vi "Joystick 0 Solenoids.vi"(8 "error in (no error)":errorcluster, 11 "button value":bool) -> (0 "error out":errorcluster)   [LabVIEW 2015]
uses:
  <vilib>/Rock Robotics/WPI/Solenoid/WPI_SolenoidValue.ctl
  <vilib>/Rock Robotics/WPI/Solenoid/Deprecated/WPI_SolenoidGetBool.vi
  <vilib>/Rock Robotics/WPI/Solenoid/WPI_SolenoidSetEnum.vi
panel:
  in  "button value 2":bool
  out "error out 2":errorcluster
  in  "error in (no error) 2":errorcluster
  # "ee"
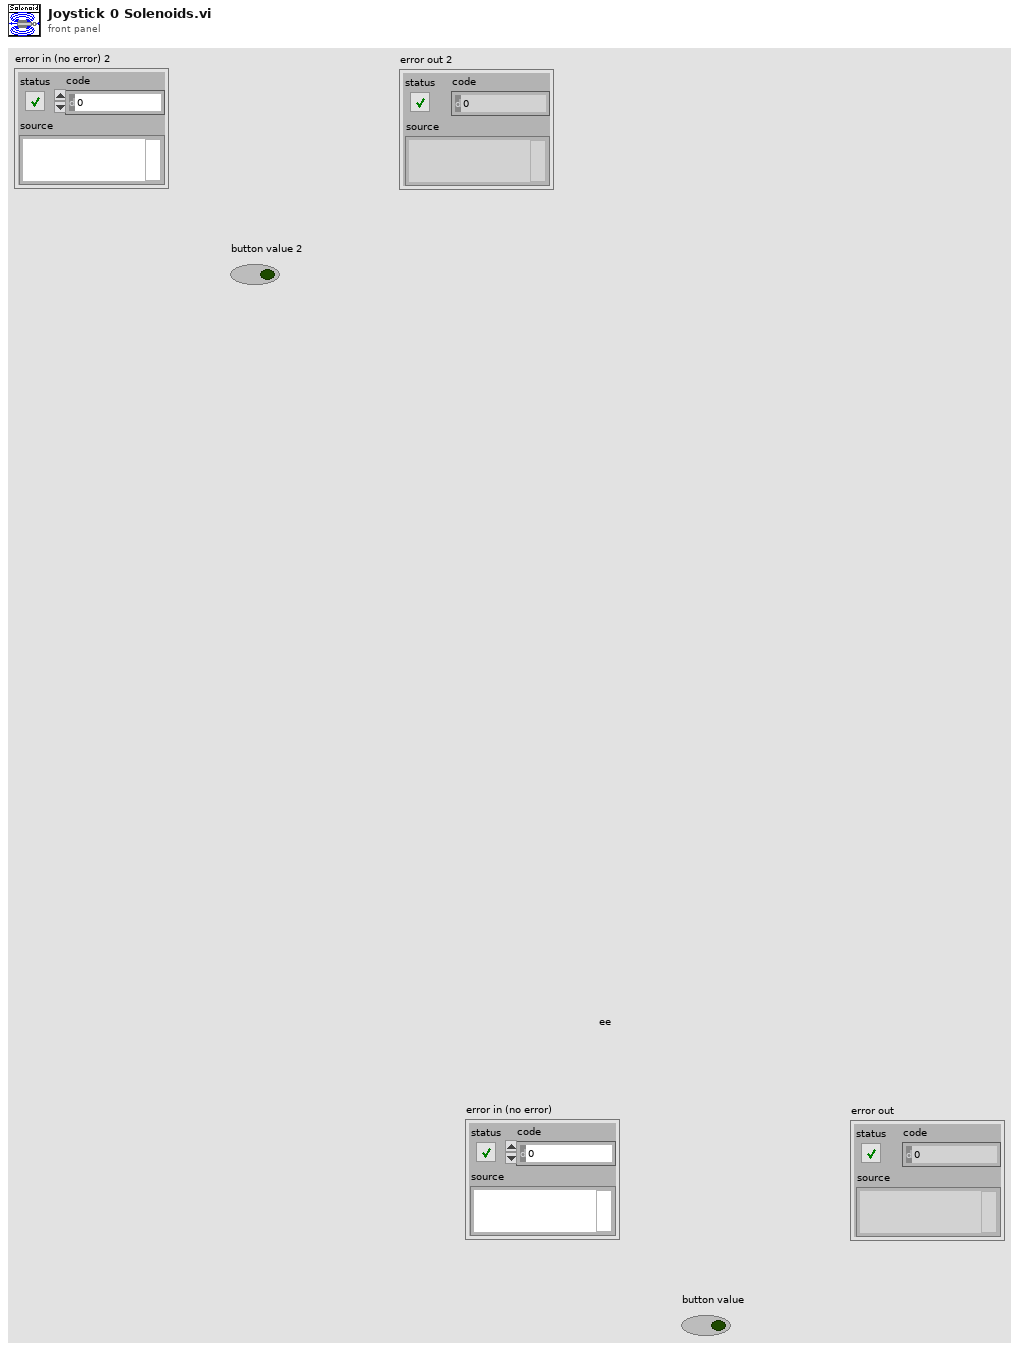
[diagram p1: front panel]
types:
  T1 = typedef "WPI_SolenoidValue.ctl" = enum16{"Off", "On", "Forward", "Reverse"}
  T2 = typedef "WPI_SolenoidDevRef.ctl" = cluster{"DevStatus":errorcluster, "Pneumatics Control Module":u8, "Forward Solenoid Channel":T3, "Reverse Solenoid Channel":T3}
  T3 = typedef "WPI_SolenoidChannel.ctl" = enum8{"Solenoid 0", "Solenoid 1", "Solenoid 2", "Solenoid 3", "Solenoid 4", "Solenoid 5", "Solenoid 6", "Solenoid 7", "Invalid"}
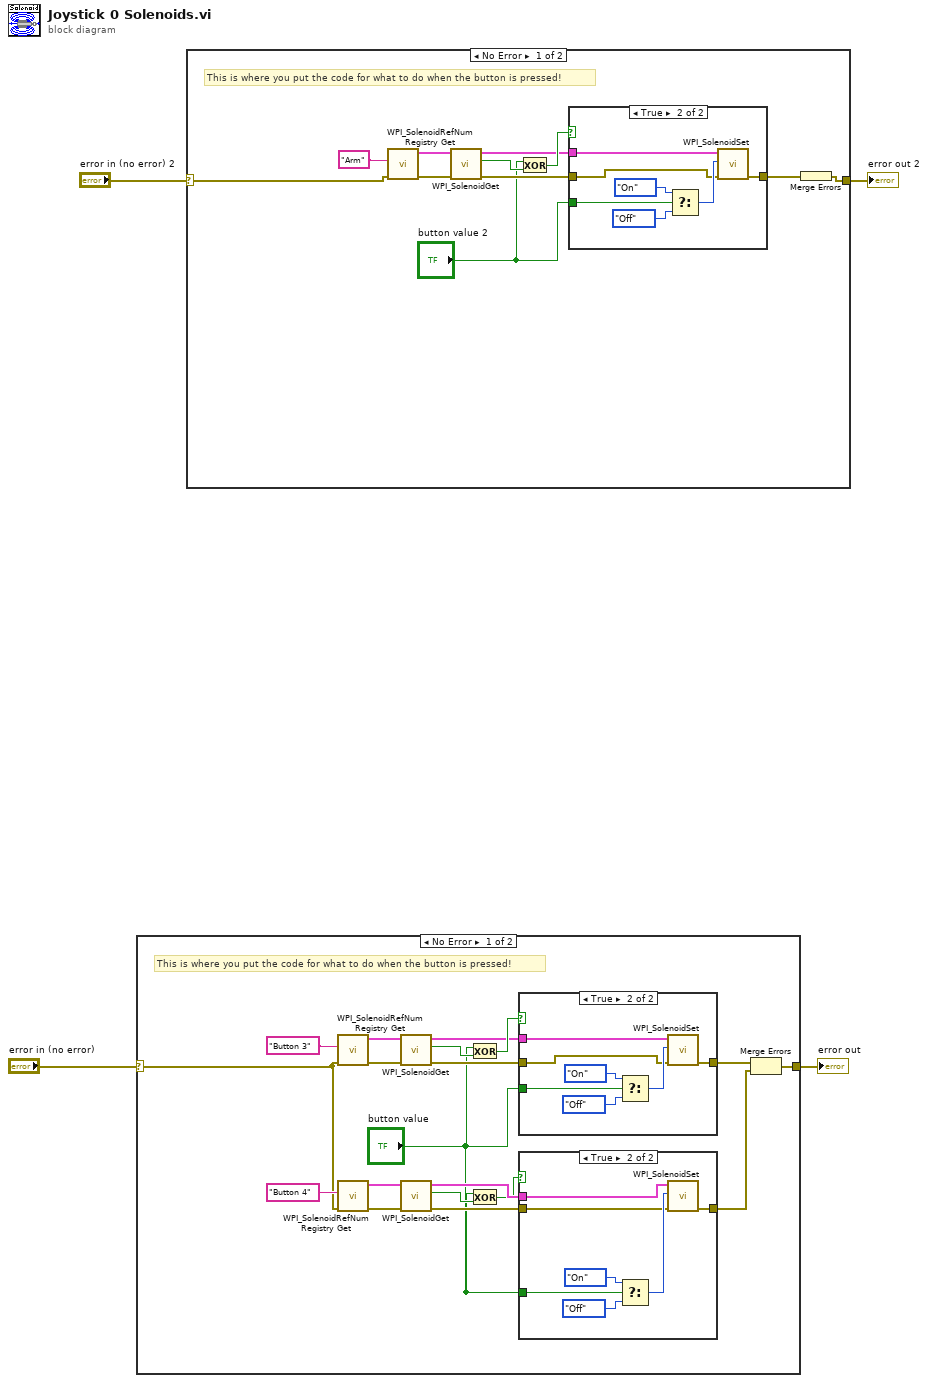
[diagram p0: block diagram]
diagram:
  n1 = case shown="No Error" "error in (no error)" {
    selector: "error in (no error)" -> [w9 w40]
    tunnel: [w6 w40] -> w3
    frame No Error {
      # "This is where you put the code for what to do when the button is pressed!"
      n2 = call <vilib>:"WPI_SolenoidRefNum Registry Get.vi"("error in (no error)"=w9, "refnum name"="Button 3") -> ("error out"=w18:errorcluster, "SolenoidDevRef"=w21:T2)  [unwired: 8 in]
      n3 = call <vilib>:"WPI_SolenoidRefNum Registry Get.vi"("error in (no error)"=w9, "refnum name"="Button 4") -> ("error out"=w15:errorcluster, "SolenoidDevRef"=w12:T2)  [unwired: 8 in]
      n4 = call-poly <vilib>:"WPI_SolenoidGet.vi"("error in (no error)"=w18, "SolenoidDevRef"=w21) -> ("error out"=w17:errorcluster, "Value"=w23:bool, "SolenoidDevRef"=w20:T2)  [unwired: 7 in]
      n5 = call-poly <vilib>:"WPI_SolenoidGet.vi"("error in (no error)"=w15, "SolenoidDevRef"=w12) -> ("error out"=w16:errorcluster, "Value"=w10:bool, "SolenoidDevRef"=w13:T2)  [unwired: 7 in]
      n6 = Exclusive Or(1:w23, 2:"button value") -> (0:w22:bool)
      n7 = Exclusive Or(1:w10, 2:"button value") -> (0:w11:bool)
      n8 = case shown="True" w22 {
        tunnel: w20 -> [_ w39]
        tunnel: "button value" -> [_ w38]
        tunnel: w17 -> [w32 w34]
        tunnel: [w32 w33] -> w7
        frame False {
        }
        frame True {
          n9 = Select(t=WPI_SolenoidValue."On" ("Value"), s=w38, f=WPI_SolenoidValue."Off" ("Value")) -> (s? t:f=w35:T1)
          n10 = call-poly <vilib>:"WPI_SolenoidSet.vi"("error in (no error)"=w34, "Value"=w35, "SolenoidDevRef"=w39) -> ("error out"=w33:errorcluster)  [unwired: 7 in, 1 out]
        }
      }
      n11 = case shown="True" w11 {
        tunnel: w13 -> [_ w31]
        tunnel: "button value" -> [_ w30]
        tunnel: w16 -> [w24 w26]
        tunnel: [w24 w25] -> w8
        frame False {
        }
        frame True {
          n12 = Select(t=WPI_SolenoidValue."On" ("Value"), s=w30, f=WPI_SolenoidValue."Off" ("Value")) -> (s? t:f=w27:T1)
          n13 = call-poly <vilib>:"WPI_SolenoidSet.vi"("error in (no error)"=w26, "Value"=w27, "SolenoidDevRef"=w31) -> ("error out"=w25:errorcluster)  [unwired: 7 in, 1 out]
        }
      }
      n14 = Merge Errors(w7, w8) -> (w6:errorcluster)
    }
    frame Error {
      # "This is what to do if there is an error.  Usually it is nothing."
    }
  }
  "error out" <- w3
  n15 = case shown="No Error" "error in (no error) 2" {
    selector: "error in (no error) 2" -> [w44 w60]
    tunnel: [w42 w60] -> w1
    frame No Error {
      # "This is where you put the code for what to do when the button is pressed!"
      n16 = call <vilib>:"WPI_SolenoidRefNum Registry Get.vi"("error in (no error)"=w44, "refnum name"="Arm") -> ("error out"=w46:errorcluster, "SolenoidDevRef"=w49:T2)  [unwired: 8 in]
      n17 = call-poly <vilib>:"WPI_SolenoidGet.vi"("error in (no error)"=w46, "SolenoidDevRef"=w49) -> ("error out"=w45:errorcluster, "Value"=w51:bool, "SolenoidDevRef"=w48:T2)  [unwired: 7 in]
      n18 = Exclusive Or(1:w51, 2:"button value 2") -> (0:w50:bool)
      n19 = case shown="True" w50 {
        tunnel: w48 -> [_ w59]
        tunnel: "button value 2" -> [_ w58]
        tunnel: w45 -> [w52 w54]
        tunnel: [w52 w53] -> w43
        frame False {
        }
        frame True {
          n20 = Select(t=WPI_SolenoidValue."On" ("Value"), s=w58, f=WPI_SolenoidValue."Off" ("Value")) -> (s? t:f=w55:T1)
          n21 = call-poly <vilib>:"WPI_SolenoidSet.vi"("error in (no error)"=w54, "Value"=w55, "SolenoidDevRef"=w59) -> ("error out"=w53:errorcluster)  [unwired: 7 in, 1 out]
        }
      }
      n22 = Merge Errors(w43) -> (w42:errorcluster)
    }
    frame Error {
      # "This is what to do if there is an error.  Usually it is nothing."
    }
  }
  "error out 2" <- w1
